vi "IdxToAccIdx.vi"(0 "Idx":u8) -> (7 "Acc. Idx":u8)   [LabVIEW 2019]
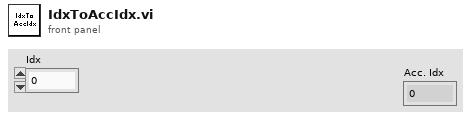
[diagram p1: front panel]
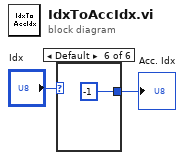
[diagram p0: block diagram]
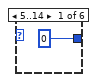
[diagram p2: hidden frame]
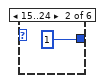
[diagram p3: hidden frame]
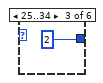
[diagram p4: hidden frame]
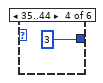
[diagram p5: hidden frame]
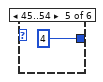
[diagram p6: hidden frame]
diagram:
  n1 = case shown="Default" "Idx" {
    tunnel: [0 1 2 3 4 -1] -> w1
    frame 5..14 {
    }
    frame 15..24 {
    }
    frame 25..34 {
    }
    frame 35..44 {
    }
    frame 45..54 {
    }
    frame Default {
    }
  }
  "Acc. Idx" <- w1
